vi "Generate Unique File Path (SubVI).vi"(9 "Measurement Name":string, 10 "file path":path, 11 "Data Folder":path) -> (0 "error out":errorcluster, 3 "appended path":path)   [LabVIEW 2020, in "FileIO.lvlib"]
uses:
  FileIO.lvlib
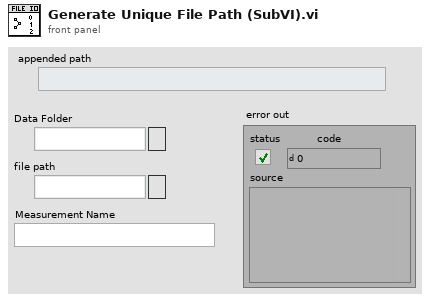
[diagram p1: front panel]
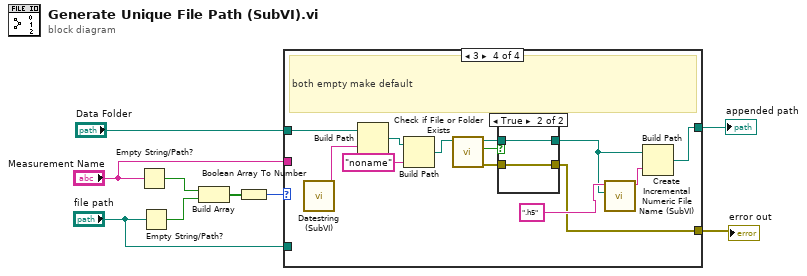
[diagram p0: block diagram]
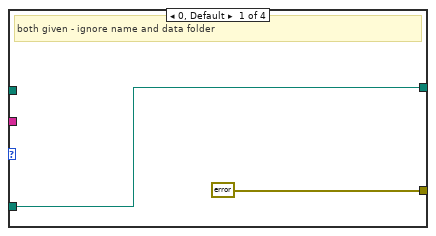
[diagram p2: hidden frame]
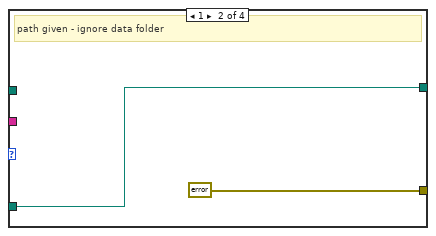
[diagram p3: hidden frame]
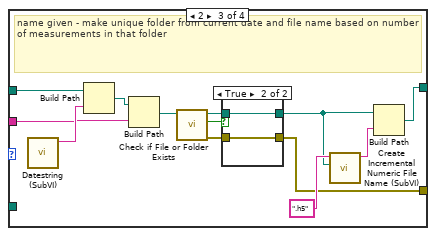
[diagram p4: hidden frame]
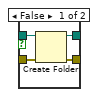
[diagram p5: hidden frame]
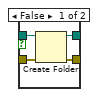
[diagram p6: hidden frame]
diagram:
  n1 = Empty String/Path?(string/path="Measurement Name") -> (empty?=w9:bool)
  n2 = Empty String/Path?(string/path="file path") -> (empty?=w8:bool)
  n3 = Build Array(w9, w8) -> (w7:bool[])
  n4 = Boolean Array To Number(Boolean array=w7) -> (number=w6:u32)
  n5 = case shown="3" w6 {
    tunnel: "file path" -> [w10 w13 _ _]
    tunnel: "Measurement Name" -> [_ _ w23 _]
    tunnel: "Data Folder" -> [_ _ w26 w45]
    tunnel: [errorcluster {"status"=FALSE, "code"=0, "source"=""} ("error out") errorcluster {"status"=FALSE, "code"=0, "source"=""} ("error out") w18 w33] -> w2
    tunnel: [w10 w13 w22 w42] -> w1
    frame 0, Default {
      # "both given - ignore name and data folder"
    }
    frame 1 {
      # "path given - ignore data folder"
    }
    frame 2 {
      # "name given - make unique folder from current date and file name based on number of measurements in that folder"
      n6 = call "Datestring (SubVI).vi"() -> ("datestring"=w25:string)  [unwired: 11 in]
      n7 = Build Path(base path=w26, name or relative path=w25) -> (appended path=w24:path)
      n8 = Build Path(base path=w24, name or relative path=w23) -> (appended path=w17:path)
      n9 = call <vilib>:"Check if File or Folder Exists.vi"("path"=w17) -> ("error out"=w15:errorcluster, "file or folder exists?"=w14:bool, "dup path"=w16:path)  [unwired: 8 in]
      n10 = case shown="True" w14 {
        tunnel: [w30 w31] -> w19
        tunnel: [w29 w32] -> w18
        tunnel: w16 -> [w28 w31]
        tunnel: w15 -> [w27 w32]
        frame False {
          n11 = Create Folder(path (use dialog)=w28, error in=w27) -> (created path=w30:path, error out=w29:errorcluster)  [unwired: 1 in, 1 out]
        }
        frame True {
        }
      }
      n12 = call "Create Incremental Numeric File Name (SubVI).vi"("folder"=w19, "file extension"=".h5" ("name or relative path")) -> ("String"=w20:string)  [unwired: 9 in]
      n13 = Build Path(base path=w19, name or relative path=w20) -> (appended path=w22:path)
    }
    frame 3 {
      # "both empty make default"
      n14 = call "Datestring (SubVI).vi"() -> ("datestring"=w41:string)  [unwired: 11 in]
      n15 = Build Path(base path=w45, name or relative path=w41) -> (appended path=w44:path)
      n16 = Build Path(base path=w44, name or relative path="noname") -> (appended path=w35:path)
      n17 = call <vilib>:"Check if File or Folder Exists.vi"("path"=w35) -> ("error out"=w37:errorcluster, "file or folder exists?"=w36:bool, "dup path"=w38:path)  [unwired: 8 in]
      n18 = case shown="True" w36 {
        tunnel: [w49 w50] -> w34
        tunnel: [w48 w51] -> w33
        tunnel: w38 -> [w47 w50]
        tunnel: w37 -> [w46 w51]
        frame False {
          n19 = Create Folder(path (use dialog)=w47, error in=w46) -> (created path=w49:path, error out=w48:errorcluster)  [unwired: 1 in, 1 out]
        }
        frame True {
        }
      }
      n20 = call "Create Incremental Numeric File Name (SubVI).vi"("folder"=w34, "file extension"=".h5" ("name or relative path")) -> ("String"=w39:string)  [unwired: 9 in]
      n21 = Build Path(base path=w34, name or relative path=w39) -> (appended path=w42:path)
    }
  }
  "appended path" <- w1
  "error out" <- w2
